vi "Optimal FIR Filter.vi"() -> ()   [LabVIEW 2023]
doc: "Demonstrates how to solve for an optimal FIR filter using the Parks McClellan method, and the linear programming method."
uses:
  <vilib>/Utility/error.llb/DialogType.ctl
  <vilib>/Analysis/1siggen.llb/Ramp Pattern by Samples.vi
  <vilib>/Analysis/NI_AALBase.lvlib
panel:
  out "Error Status":bool
  out "message":string
  out "XY Graph":cluster{dbl[], dbl[]}[](graph)
  in  "Band Parameters":T1(array[cluster])=[{"Amplitude"=2.0, "Lower Frequency"=0.0, "Upper Frequency"=0.1, "weighted ripple"=1.0}, {"Amplitude"=0.0, "Lower Frequency"=0.2, "Upper Frequency"=0.25, "weighted ripple"=1.0}, {"Amplitude"=1.0, "Lower Frequency"=0.3, "Upper Frequency"=0.5, "weighted ripple"=1.0}] {"weighted ripple" scale=0.0..1.0; "Upper Frequency" scale=0.0..0.5; "Lower Frequency" scale=0.0..0.5; "Amplitude" scale=0.0..3.0}
  in  "Stop":bool
  in  "Order":i32=9
  # "Overview: Compares Parks-McClellan and Linear Programming FIR filter designs.\nRequirements: LabVIEW Full Development System\nInstructions:\n1. Run the VI.\n2. Change the Band Parameters. Note that the upper frequency of one band must be lower than the lower frequency of the next band.\n3. Click Stop to stop the VI."
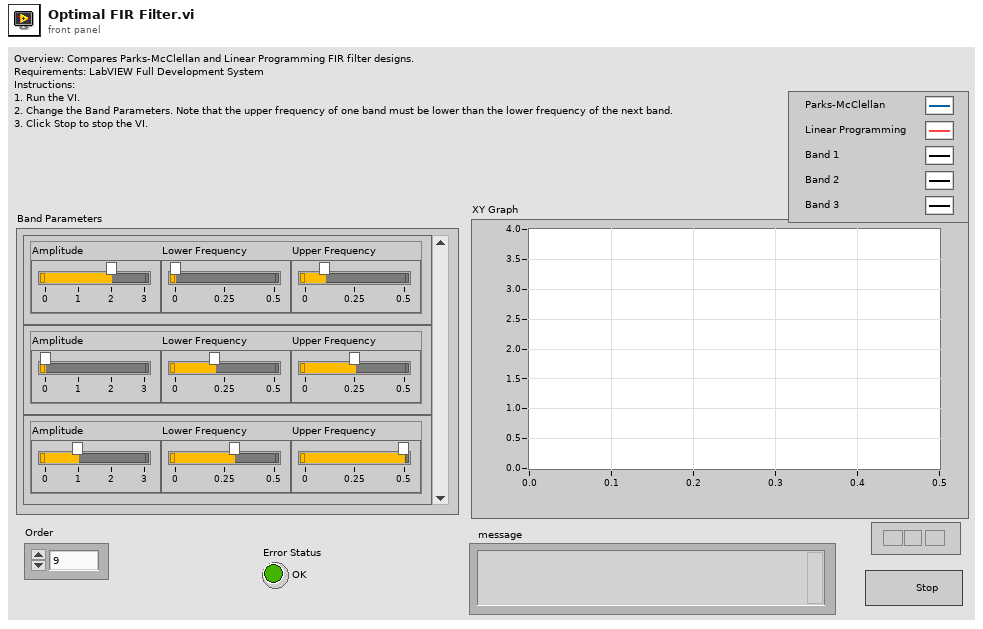
[diagram p1: front panel]
types:
  T1 = cluster{"Amplitude":dbl, "Lower Frequency":dbl, "Upper Frequency":dbl, "weighted ripple":dbl}[]
  T2 = typedef "DialogType.ctl" = u16
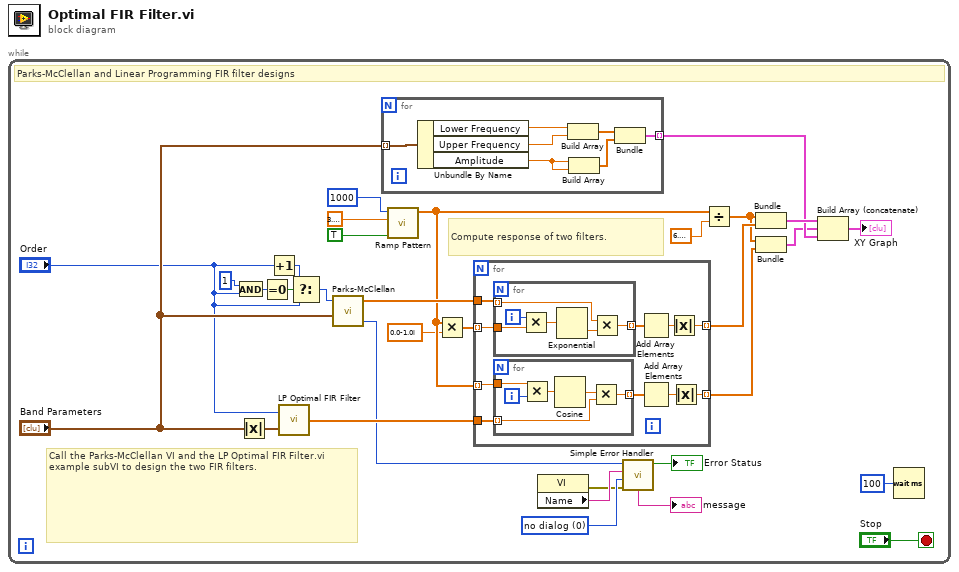
[diagram p0: block diagram]
diagram:
  n1 = while {
    stop <- "Stop" stop-if-true
    w9 = T2 0 items=["no dialog", "OK message", "continue or stop message", "OK message + warnings", "continue/stop + warnings"] ("type of dialog (OK msg:1)")
    # "Compute response of two filters."
    # "Call the Parks-McClellan VI and the LP Optimal FIR Filter.vi example subVI to design the two FIR filters."
    # "Parks-McClellan and Linear Programming FIR filter designs"
    n2 = And(x=1, y="Order") -> (x .and. y?=w21:i32)
    n3 = Absolute Value(x="Band Parameters") -> (abs(x)=w13:T1)
    n4 = Equal To 0?(x=w21) -> (x = 0?=w20:bool)
    n5 = Increment(x="Order") -> (x+1=w19:i32)
    n6 = call "LP Optimal FIR Filter.vi"("Band Parameters"=w13, "# of taps"="Order") -> ("h new"=w27:dbl[])
    n7 = Select(t=w19, s=w20, f="Order") -> (s? t:f=w18:i32)
    n8 = call <vilib>:"Parks-McClellan.vi"("Band Parameters"="Band Parameters", "# of taps"=w18) -> ("error"=w6:i32, "h"=w31:dbl[])  [unwired: 2 in, 1 out]
    n9 = for {
      tunnel: "Band Parameters" -> [w39] mode=indexing
      tunnel: [w34] -> w12 mode=indexing
      n10 = Unbundle By Name(w39) -> ("Lower Frequency"=w38:dbl, "Upper Frequency"=w37:dbl, "Amplitude"=w33:dbl)
      n11 = Build Array(w38, w37) -> (w36:dbl[])
      n12 = Build Array(w33, w33) -> (w35:dbl[])
      n13 = Bundle(w36, w35) -> (w34:cluster{dbl[], dbl[]})  [unwired: 1 in]
    }
    n14 = call-poly <vilib>:"Ramp Pattern.vi"("exclude end?"=TRUE, "end"=3.141592653589793, "samples"=1000) -> ("Ramp Pattern"=w15:dbl[])  [unwired: 7 in, 1 out]
    n15 = Multiply(x=w15, y=cdb 0.0-1.0i) -> (x*y=w29:cdb[])
    n16 = for {
      tunnel: w29 -> [w44] mode=indexing
      tunnel: w31 -> [w49]
      tunnel: [w41] -> w30 mode=indexing
      tunnel: w27 -> [w46]
      tunnel: [w40] -> w25 mode=indexing
      tunnel: w15 -> [w43] mode=indexing
      n17 = for {
        tunnel: w49 -> [w59] mode=indexing
        tunnel: [w58] -> w48 mode=indexing
        tunnel: w44 -> [w56]
        i -> [w61]
        n18 = Multiply(x=w61, y=w56) -> (x*y=w60:cdb)
        n19 = Exponential(1:w60) -> (0:w57:cdb)
        n20 = Multiply(x=w59, y=w57) -> (x*y=w58:cdb)
      }
      n21 = for {
        tunnel: [w54] -> w45 mode=indexing
        tunnel: w43 -> [w53]
        tunnel: w46 -> [w52] mode=indexing
        i -> [w55]
        n22 = Multiply(x=w53, y=w55) -> (x*y=w50:dbl)
        n23 = Cosine(x=w50) -> (cos(x)=w51:dbl)
        n24 = Multiply(x=w51, y=w52) -> (x*y=w54:dbl)
      }
      n25 = Add Array Elements(numeric array=w48) -> (sum=w47:cdb)
      n26 = Add Array Elements(numeric array=w45) -> (sum=w42:dbl)
      n27 = Absolute Value(x=w47) -> (abs(x)=w41:dbl)
      n28 = Absolute Value(x=w42) -> (abs(x)=w40:dbl)
    }
    n29 = property class="VI"() -> (error out=w2:errorcluster, "Name"=w3:string)  [unwired: 2 in, 1 out]
    n30 = call <vilib>:"Simple Error Handler.vi"("error code (no error:0)"=w6, "error source (\" \")"=w3, "type of dialog (OK msg:1)"=w9, "error in (no error)"=w2) -> ("error?"=→"Error Status":bool, "message"=→"message":string)  [unwired: 1 in, 3 out]
    n31 = Divide(x=w15, y=6.283185307179586) -> (x/y=w26:dbl[])
    n32 = Bundle(w26, w30) -> (w24:cluster{dbl[], dbl[]})  [unwired: 1 in]
    n33 = Bundle(w26, w25) -> (w11:cluster{dbl[], dbl[]})  [unwired: 1 in]
    n34 = Build Array (concatenate)(w24, w11, w12) -> (→"XY Graph":cluster{dbl[], dbl[]}[])
    n35 = Wait (ms)(milliseconds to wait=u32 100) -> ()  [unwired: 1 out]
  }
